vi "FTQF.vi"(6 "delay (500 ms) after write":u32=500, 7 "Frequency GHz":string, 8 "error in (no error)":errorcluster, 11 "VISA resource name":refnum<visa-resource-name>="COM11") -> (0 "error out":errorcluster, 3 "VISA resource name out":refnum<visa-resource-name>, 5 "Response":string)   [LabVIEW 2020]
doc: "This example performs a serial port write and a serial port read. The parameters set for the serial port must match the parameters of the connected instrument or device. The VISA Configure Serial Port VI sets the configuration parameters. The front panel displays the controls used to configure the basic parameters, such as baud rate, data bits, and parity. The VI passes the VISA resource name to other VIs that perform operations on that VISA resource. The VISA Write function sends a command to the serial device and the VISA Read function returns data based on the command. The VISA Close function then closes the reference to the serial device. It is important to close the reference; otherwise, further communication through that port might not be possible."
panel:
  out "concatenated string":string
  # "Title:  FTQT \nOverview:  Use the VISA functions to send a single FT command, followed immedeatly by the query QF command and read the response  from the  serial instrument 3 times to get the read a response of the QF command.\nRequirements: NI-VISA Driver\nInstructions:\n1. This VI excpects the caller to corretly open and configure the VISA serial settings the same as the Putty stand alone.\n2. Ensure the resource specified by the VISA resource name is a valid serial device.\n3. If the DUT accepts the FT frequency command, this VI will return the QF with the same frequecy\n4. The caller should then compare the QF Response against the FT frequency."
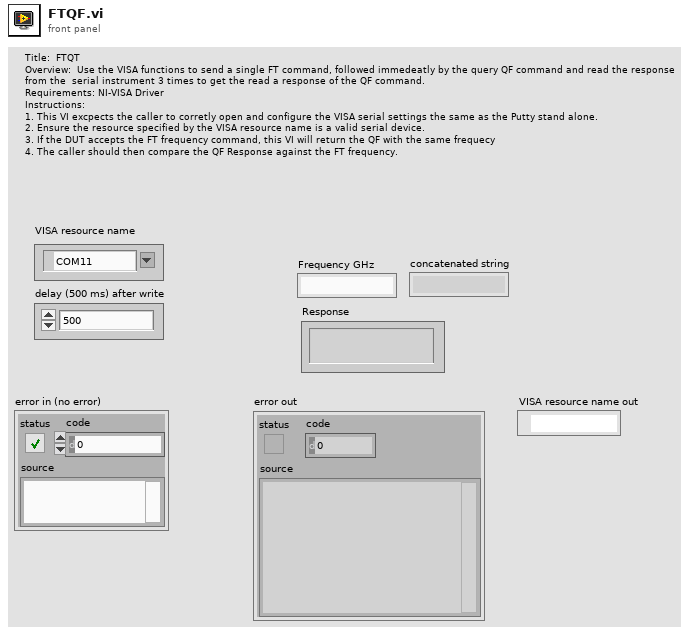
[diagram p1: front panel]
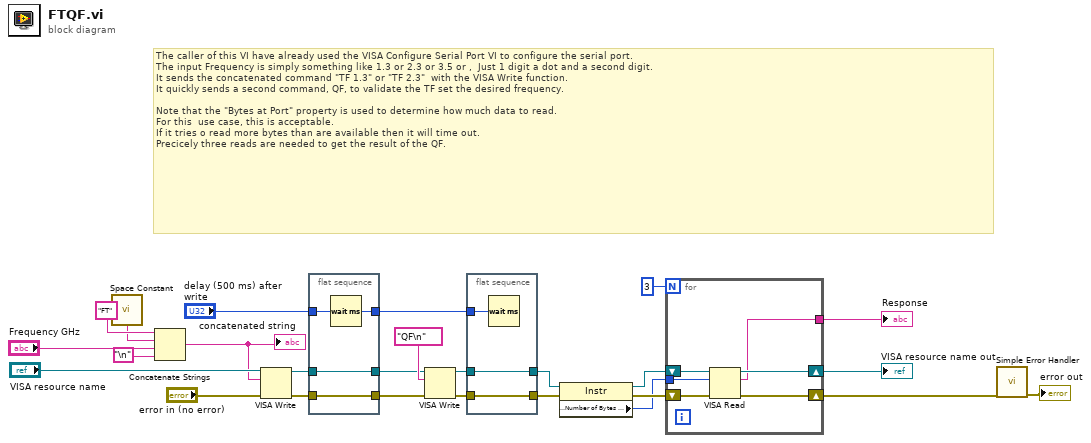
[diagram p0: block diagram]
diagram:
  # "The caller of this VI have already used the VISA Configure Serial Port VI to configure the serial port. \nThe input Frequency is simply something like 1.3 or 2.3 or 3.5 or ,  Just 1 digit a dot and a second digit.\nIt sends the concatenated command \"TF 1.3\" or \"TF 2.3\"  with the VISA Write function.\nIt quickly sends a second command, QF, to validate the TF set the desired frequency. \n\nNote that the \"Bytes at Port\" property is used to determine how much data to read. \nFor this  use case, this is acceptable. \nIf it tries o read more bytes than are available then it will time out.\nPrecicely three reads are needed to get the result of the QF."
  n1 = call <vilib>:"Space Constant.vi"() -> ("String"=w8:string)
  n2 = Concatenate Strings("FT" ("string"), w8, "Frequency GHz", "\n") -> (w10:string)
  "concatenated string" <- w10
  n3 = VISA Write(VISA resource name="VISA resource name", write buffer=w10, error in (no error)="error in (no error)") -> (VISA resource name out=w12:refnum<visa-resource-name>, error out=w11:errorcluster)  [unwired: 1 out]
  n4 = flat-sequence {
    tunnel: w11 -> [w29]
    tunnel: [w29] -> w5
    tunnel: w12 -> [w28]
    tunnel: [w28] -> w6
    tunnel: "delay (500 ms) after write" -> [w27]
    tunnel: [w27] -> w13
    frame #0 {
      n5 = Wait (ms)(milliseconds to wait=w27) -> ()  [unwired: 1 out]
    }
  }
  n6 = VISA Write(VISA resource name=w6, write buffer="QF\n" ("Command"), error in (no error)=w5) -> (VISA resource name out=w22:refnum<visa-resource-name>, error out=w24:errorcluster)  [unwired: 1 out]
  n7 = flat-sequence {
    tunnel: w24 -> [w31]
    tunnel: [w31] -> w23
    tunnel: w22 -> [w30]
    tunnel: [w30] -> w21
    tunnel: w13 -> [w32]
    frame #0 {
      n8 = Wait (ms)(milliseconds to wait=w32) -> ()  [unwired: 1 out]
    }
  }
  n9 = property class="Instr"(reference=w21, error in=w23) -> (reference out=w19:refnum<visa-resource-name>, error out=w18:errorcluster, "Serial Settings:Number of Bytes at Serial Port"=w17:u32)
  n10 = for {
    N: 3 ("Numeric") -> [_]
    tunnel: w17 -> [w34]
    shift-right: [w37] -> w2
    shift-left: w19 -> [w36]
    shift-right: [w38] -> w25
    shift-left: w18 -> [w35]
    tunnel: [w33] -> w16
    n11 = VISA Read(VISA resource name=w36, byte count=w34, error in (no error)=w35) -> (VISA resource name out=w37:refnum<visa-resource-name>, read buffer=w33:string, error out=w38:errorcluster)  [unwired: 1 out]
  }
  "Response" <- w16
  "VISA resource name out" <- w2
  n12 = call <vilib>:"Simple Error Handler.vi"("error in (no error)"=w25) -> ("error out"=→"error out":errorcluster)  [unwired: 1 in, 7 out]
